vi "Bad Setting Error.vi"(7 "vi name":string, 8 "error in (no error)":errorcluster, 9 "value":string, 10 "key":string, 11 "PXImc Transceiver in":refnum<class "DSF PXImc Transceiver.lvclass">=refnum) -> (0 "error out":errorcluster, 3 "PXImc Transceiver out":refnum<class "DSF PXImc Transceiver.lvclass">)   [LabVIEW 2017, in "DSF Core.lvlib" / "DSF PXImc Transceiver.lvclass"]
uses:
  DSF PXImc Transceiver.lvclass
  Errors.ctl
  <vilib>/NI/Memory Manager/Static Errors.lvlib
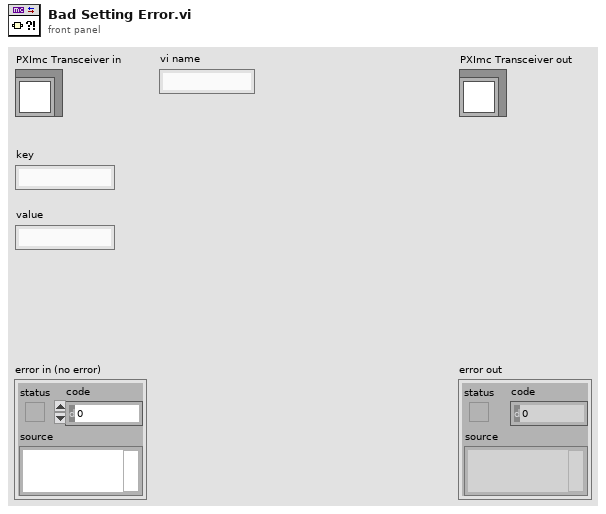
[diagram p1: front panel]
types:
  T1 = typedef "DSF Core.lvlib/DSF PXImc Transceiver.lvclass/Errors.ctl" = enum8{"Bad Setting", "Duplicate Stream ID"}
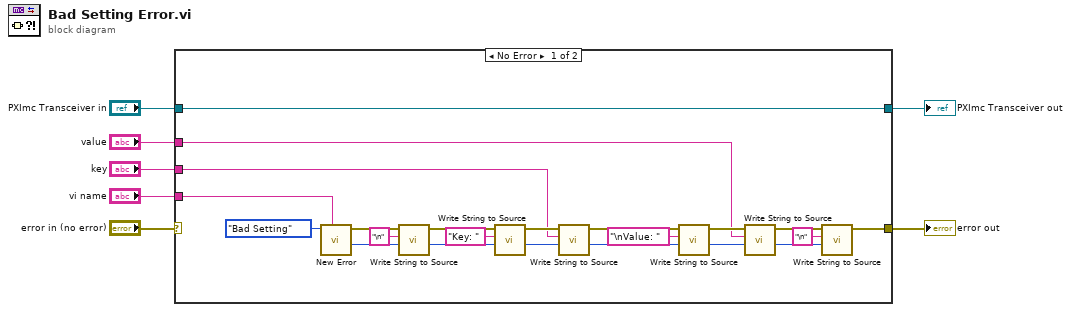
[diagram p0: block diagram]
diagram:
  n1 = case shown="No Error" "error in (no error)" {
    selector: "error in (no error)" -> [_ w31]
    tunnel: [w19 w31] -> w6
    tunnel: [w29 w30] -> w4
    tunnel: "PXImc Transceiver in" -> [w29 w30]
    tunnel: "vi name" -> [w27 _]
    tunnel: "value" -> [w11 _]
    tunnel: "key" -> [w16 _]
    frame No Error {
      n2 = call "New Error.vi"("vi name"=w27, "error"=Errors."Bad Setting") -> ("initial offset"=w8:i32, "error"=w26:errorcluster)  [unwired: 8 in]
      n3 = call <vilib>:"Write String to Source.vi"("offset"=w8, "string"="\n", "error in"=w26) -> ("new offset"=w24:i32, "error out"=w23:errorcluster)  [unwired: 7 in]
      n4 = call <vilib>:"Write String to Source.vi"("offset"=w24, "string"="Key: ", "error in"=w23) -> ("new offset"=w17:i32, "error out"=w18:errorcluster)  [unwired: 7 in]
      n5 = call <vilib>:"Write String to Source.vi"("offset"=w17, "string"=w16, "error in"=w18) -> ("new offset"=w15:i32, "error out"=w14:errorcluster)  [unwired: 7 in]
      n6 = call <vilib>:"Write String to Source.vi"("offset"=w15, "string"="\nValue: ", "error in"=w14) -> ("new offset"=w12:i32, "error out"=w13:errorcluster)  [unwired: 7 in]
      n7 = call <vilib>:"Write String to Source.vi"("offset"=w12, "string"=w11, "error in"=w13) -> ("new offset"=w9:i32, "error out"=w10:errorcluster)  [unwired: 7 in]
      n8 = call <vilib>:"Write String to Source.vi"("offset"=w9, "string"="\n", "error in"=w10) -> ("error out"=w19:errorcluster)  [unwired: 7 in, 1 out]
    }
    frame Error {
    }
  }
  "error out" <- w6
  "PXImc Transceiver out" <- w4
